vi "GetListing.vi"(8 "error in (no error)":errorcluster, 9 "Reset?":bool, 10 "Server":path) -> (0 "error out":errorcluster, 1 "Found":bool, 3 "VI out":refnum<vi>)   [LabVIEW 2020]
panel:
  out "Array":T1(array[cluster])
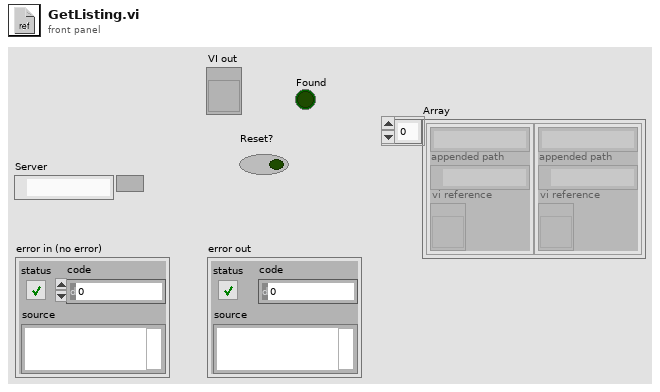
[diagram p1: front panel]
types:
  T1 = cluster{string, "appended path":path, "vi reference":refnum<vi>}[]
  T2 = cluster{string, "appended path":path, "vi reference":refnum<vi>}
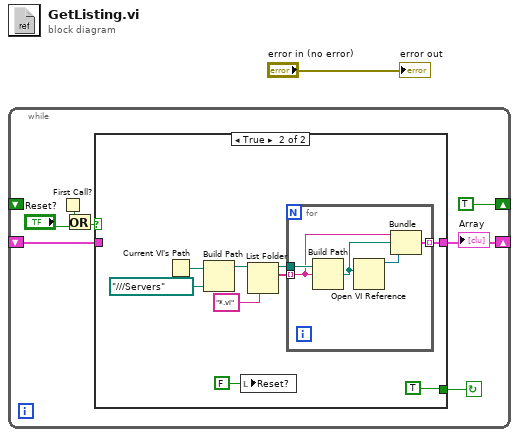
[diagram p0: block diagram]
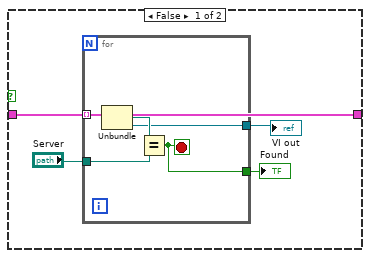
[diagram p2: hidden frame]
diagram:
  n1 = while {
    shift-right: [TRUE] -> _
    shift-left: _ -> [_]
    shift-right: [w7] -> _
    shift-left: _ -> [w6]
    stop <- w5 continue-if-true
    n2 = First Call?() -> (First Call?: T/F=w4:bool)
    n3 = Or(x=w4, y="Reset?") -> (x .or. y?=w3:bool)
    n4 = case shown="True" w3 {
      tunnel: [w10 w20] -> w7
      tunnel: w6 -> [w10 _]
      tunnel: [_ TRUE] -> w5
      frame False {
        n5 = for {
          tunnel: w10 -> [w17] mode=indexing
          tunnel: "Server" -> [w15]
          tunnel: [w14] -> w11
          tunnel: [w13] -> w9
          stop <- w13 stop-if-true
          n6 = Unbundle(w17) -> ("appended path"=w16:path, "vi reference"=w14:refnum<vi>)  [unwired: 1 out]
          n7 = Equal?(x=w16, y=w15) -> (x = y?=w13:bool)
        }
        "VI out" <- w11
        "Found" <- w9
      }
      frame True {
        n8 = Current VI's Path() -> (path=w25:path)
        n9 = Build Path(base path=w25, name or relative path=path "../../../Servers") -> (appended path=w26:path)
        n10 = local write "Reset?"(FALSE ("Reset?")) -> ()
        n11 = List Folder(path=w26, pattern="*.vi") -> (path out=w21:path, filenames=w22:string[])  [unwired: 2 in, 2 out]
        n12 = for {
          tunnel: w22 -> [w30] mode=indexing
          tunnel: w21 -> [w31]
          tunnel: [w27] -> w20 mode=indexing
          n13 = Build Path(base path=w31, name or relative path=w30) -> (appended path=w29:path)
          n14 = Open VI Reference(vi path=w29) -> (vi reference=w28:refnum<vi>)  [unwired: 5 in, 1 out]
          n15 = Bundle(w30, "appended path"=w29, "vi reference"=w28) -> (w27:T2)  [unwired: 1 in]
        }
      }
    }
    "Array" <- w7
  }
  "error out" <- "error in (no error)"
